vi "run.fpga.test.vi"(8 "error in (no error)":errorcluster, 10 "Test.Parms":T1, 11 "Refnum in":refnum<k20>) -> (0 "error out":errorcluster, 2 "Fpga\nData.out":u64[](array[numeric]), 3 "Refnum out":refnum<k20>)   [LabVIEW 2021]
uses:
  <vilib>/Utility/error.llb/Error Cluster From Error Code.vi
  <vilib>/rvi/errors/niLvFpgaAdjustHostInterfaceError.vi
  <vilib>/rvi/interface/nirviMethod/nirviMethod.xnode
  <vilib>/FPGAPlugInAG/Dynamic/niLvFpga_ReadFifo_Dynamic.vi
  <vilib>/rvi/errors/niLvFpgaMergeErrorWithErrorCode.vi
  <vilib>/FPGAPlugInAG/Dynamic/niLvFpga_WriteFifo_Dynamic.vi
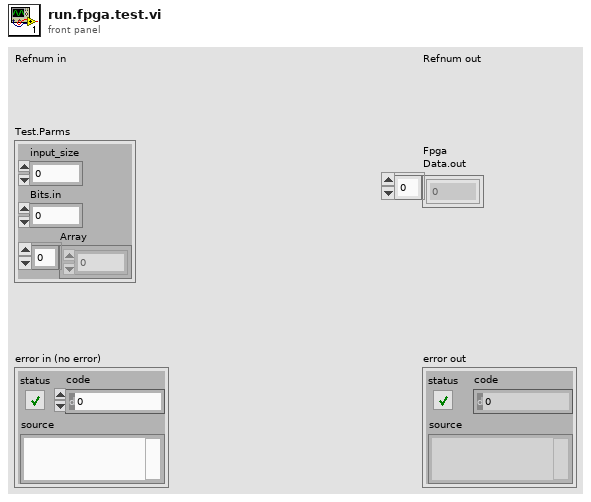
[diagram p1: front panel]
types:
  T1 = cluster{"input_size":i32, "Bits.in":u32, "Array":u64[]}
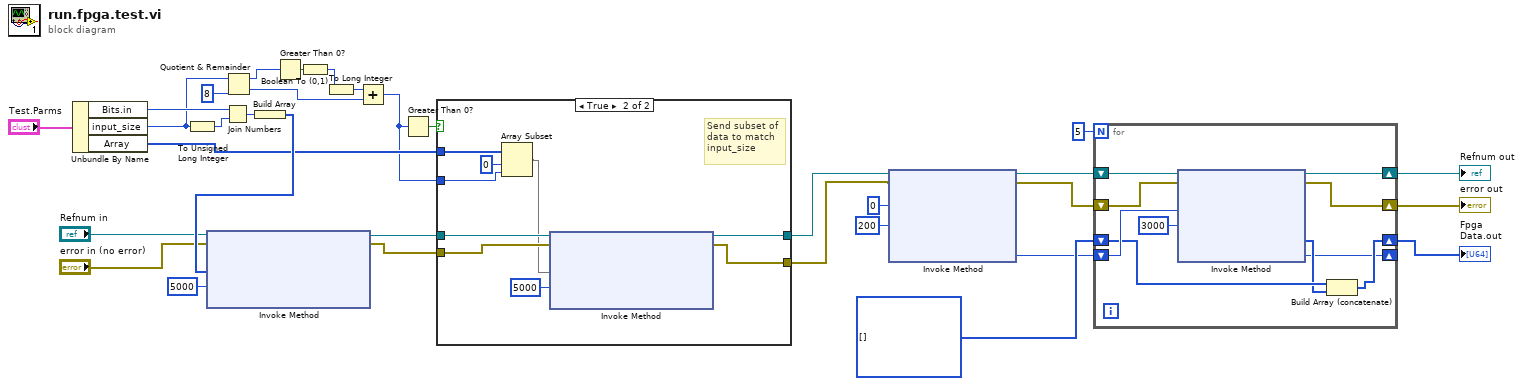
[diagram p0: block diagram]
diagram:
  n1 = Unbundle By Name("Test.Parms") -> ("Bits.in"=w11:u32, "input_size"=w4:i32, "Array"=w12:u64[])
  n2 = To Unsigned Long Integer(number=w4) -> (unsigned 32bit integer=w5:u32)
  n3 = Join Numbers(hi=w11, lo=w5) -> ((hi.lo)=w19:u64)
  n4 = Quotient & Remainder(x=w4, y=8) -> (x-y*floor(x/y)=w7:i32, floor(x/y)=w9:i32)
  n5 = Build Array(w19) -> (w16:u64[])
  n6 = xnode "Invoke Method"("FPGA VI Reference In"="Refnum in", "error in"="error in (no error)", "Data"=w16, "Timeout (ms)"=5000) -> ("FPGA VI Reference Out"=w28:refnum<k20>, "error out"=w29:errorcluster)  [unwired: 1 out]
  n7 = Greater Than 0?(x=w7) -> (x > 0?=w6:bool)
  n8 = Boolean To (0,1)(Boolean=w6) -> (0, 1=w3:i16)
  n9 = To Long Integer(number=w3) -> (32bit integer=w2:i32)
  n10 = Add(x=w2, y=w9) -> (x+y=w1:i32)
  n11 = Greater Than 0?(x=w1) -> (x > 0?=w27:bool)
  n12 = case shown="True" w27 {
    tunnel: w12 -> [_ w43]
    tunnel: w28 -> [w34 w41]
    tunnel: w29 -> [w33 w40]
    tunnel: [w34 w37] -> w30
    tunnel: [w33 w36] -> w31
    tunnel: w1 -> [_ w35]
    frame False {
    }
    frame True {
      # "Send subset of\ndata to match\ninput_size"
      n13 = Array Subset(array=w43, index=0, length=w35) -> (w39:u64[])
      n14 = xnode "Invoke Method"("FPGA VI Reference In"=w41, "error in"=w40, "Data"=w39, "Timeout (ms)"=5000) -> ("FPGA VI Reference Out"=w37:refnum<k20>, "error out"=w36:errorcluster)  [unwired: 1 out]
    }
  }
  n15 = xnode "Invoke Method"("FPGA VI Reference In"=w30, "error in"=w31, "Number of Elements"=u32 0, "Timeout (ms)"=200) -> ("FPGA VI Reference Out"=w21:refnum<k20>, "error out"=w20:errorcluster, "Elements Remaining"=w23:u32)  [unwired: 1 out]
  n16 = for {
    N: 5 -> [_]
    shift-right: [w52] -> w22
    shift-left: w21 -> [w53]
    shift-right: [w51] -> w10
    shift-left: w20 -> [w50]
    shift-right: [w46] -> w24
    shift-left: u64[] [] ("Fpga\nData.out 2") -> [w47]
    shift-right: [w44] -> _
    shift-left: w23 -> [w49]
    n17 = xnode "Invoke Method"("FPGA VI Reference In"=w53, "error in"=w50, "Number of Elements"=w49, "Timeout (ms)"=3000) -> ("FPGA VI Reference Out"=w52:refnum<k20>, "error out"=w51:errorcluster, "Data"=w45:u64[], "Elements Remaining"=w44:u32)
    n18 = Build Array (concatenate)(w47, w45) -> (w46:u64[])
  }
  "Fpga\nData.out" <- w24
  "Refnum out" <- w22
  "error out" <- w10
